vi "OA Orbit Plot.vi"   [LabVIEW 2017]
doc: "Draws an orbit plot with unfiltered or filtered data on an XY graph. The unfiltered data comes from the <B>even-angle signals</B> input, and the filtered data comes from the <B>magnitudes</B> and <B>phases [phase lag]</B> inputs."
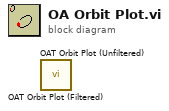
[diagram p0: block diagram]
diagram:
  n1 = call <vilib>:"OAT Orbit Plot (Filtered).vi"() -> ()  [unwired: 13 in, 3 out]
  n2 = call <vilib>:"OAT Orbit Plot (Unfiltered).vi"() -> ()  [unwired: 14 in, 2 out]
